vi "Demo_TRIGGER_SQL_DATA.vi"(4 "STATION ID_CID":string, 6 "TABLE NAME":string, 7 "BREAKDOWN ID":i32, 8 "error in (no error)":errorcluster, 9 "ID MAX":i32, 10 "Shift":i32, 11 "Refnum in":T1) -> (0 "error out":errorcluster, 3 "Refnum out":T1)   [LabVIEW 2017]
uses:
  <vilib>/addons/database/Connection.llb/Conn ObjectReference.ctl
  <vilib>/addons/database/NI_Database_API.lvlib
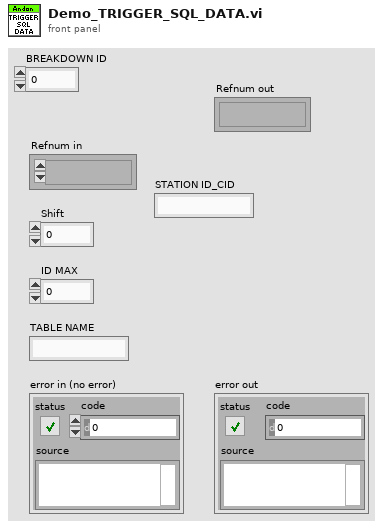
[diagram p1: front panel]
types:
  T1 = typedef "NI_Database_API.lvlib/Conn ObjectReference.ctl" = refnum<k1>
  T2 = cluster{i32, string, "STATION ID_CID":string, "Shift":i32, "date/time string":string, "Date String":string, "Date String":string, i32}
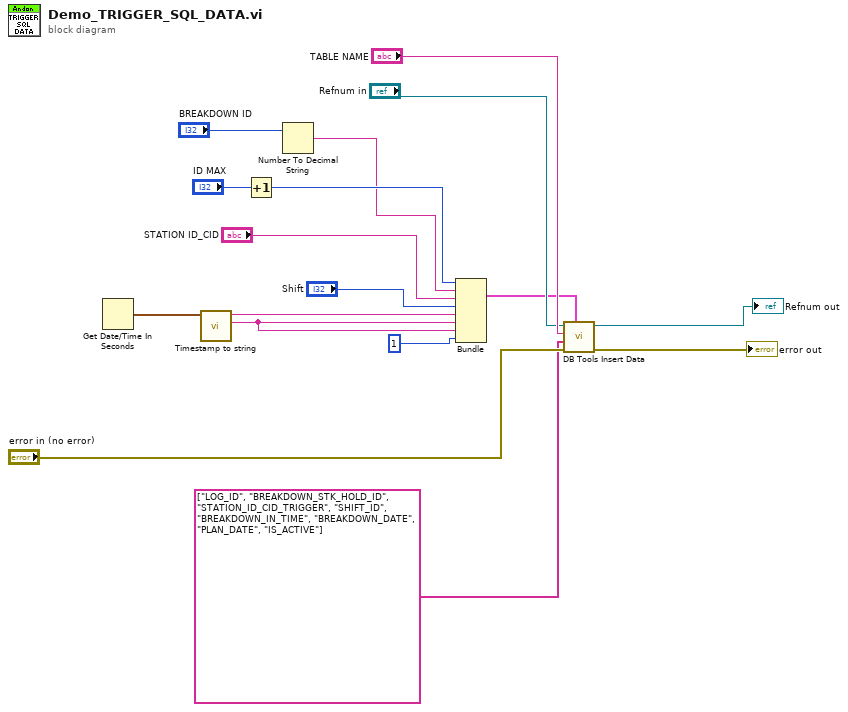
[diagram p0: block diagram]
diagram:
  n1 = Get Date/Time In Seconds() -> (seconds since 1Jan1904=w5:timestamp)
  n2 = call "Timestamp to string.vi"("time stamp"=w5) -> ("Date String"=w3:string, "date/time string"=w4:string)  [unwired: 8 in, 1 out]
  n3 = Increment(x="ID MAX") -> (x+1=w15:i32)
  n4 = Number To Decimal String(number="BREAKDOWN ID") -> (decimal integer string=w2:string)  [unwired: 1 in]
  n5 = Bundle(w15, w2, "STATION ID_CID"="STATION ID_CID", "Shift"="Shift", "date/time string"=w4, "Date String"=w3, "Date String"=w3, 1) -> (w10:T2)  [unwired: 1 in]
  n6 = call <vilib>:"DB Tools Insert Data.vi"("data"=w10, "error in (no error)"="error in (no error)", "columns"=string[] ["LOG_ID", "BREAKDOWN_STK_HOLD_ID", "STATION_ID_CID_TRIGGER", "SHIFT_ID", "BREAKDOWN_IN_TIME", "BREAKDOWN_DATE", "PLAN_DATE", "IS_ACTIVE"], "table"="TABLE NAME", "connection reference"="Refnum in") -> ("error out"=→"error out":errorcluster, "connection reference out"=→"Refnum out":T1)  [unwired: 5 in]
